vi "build matrix.vi"(9 "value":dbl, 10 "num col":i32, 11 "num row":i32) -> (3 "Array":dbl[][](array[numeric]))   [LabVIEW 2012, in "LightPipes.lvlib"]
uses:
  LightPipes.lvlib
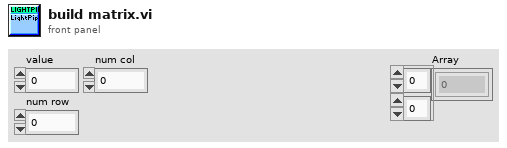
[diagram p1: front panel]
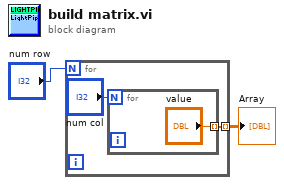
[diagram p0: block diagram]
diagram:
  n1 = for {
    N: "num row" -> [_]
    tunnel: [w4] -> w1 mode=indexing
    n2 = for {
      N: "num col" -> [_]
      tunnel: ["value"] -> w4 mode=indexing
    }
  }
  "Array" <- w1
